vi "Example LV.vi"() -> ()   [LabVIEW 2020]
uses:
  <vilib>/Math Plots/3D Math Plots/3D Scatter/3D Scatter XCtrl/3D Scatter.xctl
  <vilib>/Utility/sysdir.llb/System Directory Type.ctl
  Sources/_Helpers/Tiff Page Details.ctl
  <vilib>/Analysis/1siggen.llb/Ramp Pattern by Samples.vi
  <vilib>/Math Plots/3D Math Plots/3D Scatter/3D Scatter Datatype/Public/Plot Helper (Matrix).vi
  Sources/TIFF Writer/TIFF Writer.lvclass
  Sources/LV Tiff.lvlib
  Sources/TIFF Reader/TIFF Reader.lvclass
  <vilib>/Analysis/NI_AALBase.lvlib
  <vilib>/Math Plots/3D Math Plots/3D Scatter/3D Scatter Datatype/3D Scatter Datatype.lvclass
panel:
  out "size(s)":i32
  out "3D Scatter":refnum<class "3D Plot Datatype.lvclass">[](xcontrol)
  out "Deflate":picture
  out "JPEG":picture
  out "Raw Picture":picture
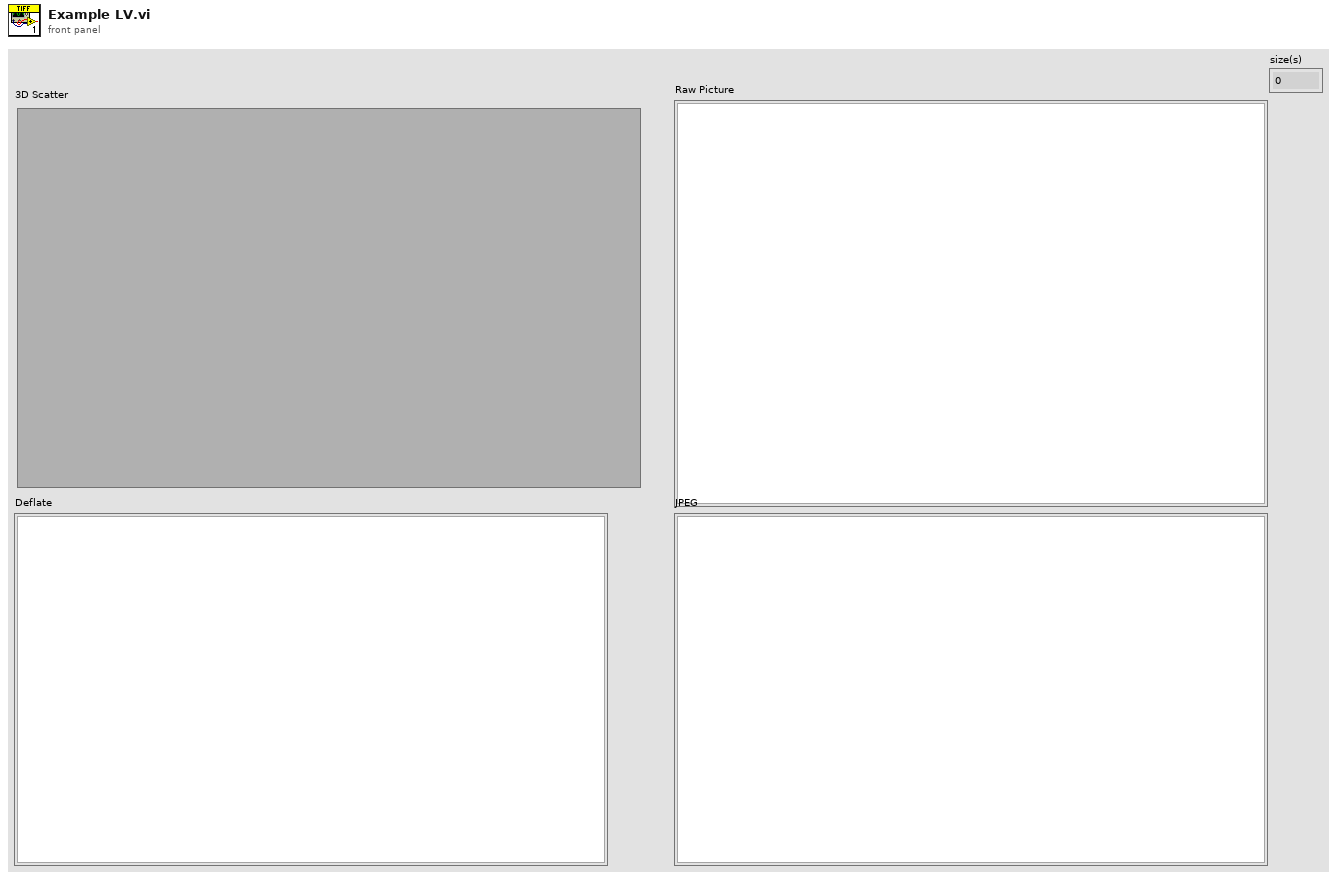
[diagram p1: front panel]
types:
  T1 = enum16{"open", "replace", "create", "open or create", "replace or create", "replace or create with confirmation"}
  T2 = typedef "System Directory Type.ctl" = i32
  T3 = typedef "imagedata.ctl" = cluster{"image type":i32, "image depth":i32, "image":u8[], "mask":u8[], "colors":u32[], "Rectangle":cluster{"left":i16, "top":i16, "right":i16, "bottom":i16}}
  T4 = typedef "LV Tiff.lvlib/Tiff Page Details.ctl" = cluster{"ImageDescription":string, "XResolution":dbl, "YResolution":dbl, "ResolutionUnit":enum16{"None", "Inch", "Centimeter"}, "PhotometricInterpretation":u16, "Compression":enum16{"None", "Deflate", "JPEG"}, "PageName":string, "DocumentName":string}
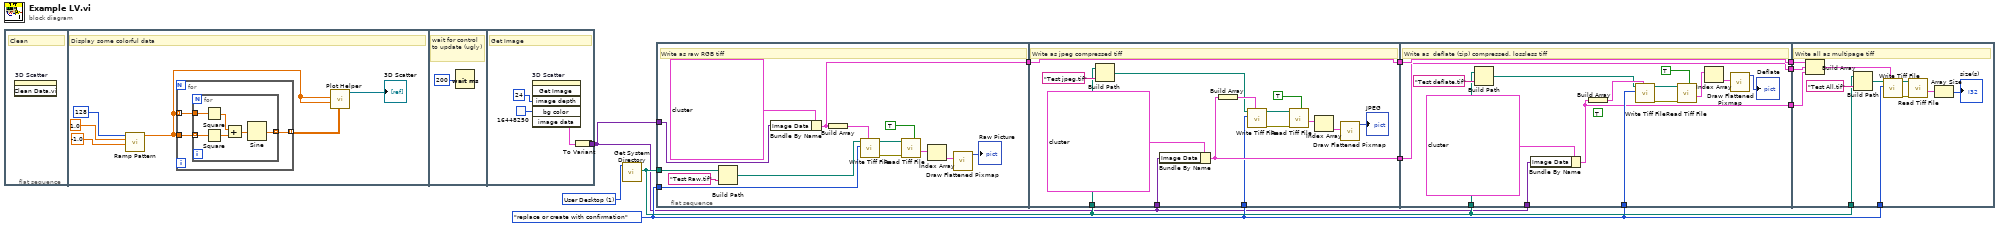
[diagram p0: block diagram]
diagram:
  w2 = T1."replace or create with confirmation" ("operation (replace)")
  w10 = T2 1 items=["User Home"=0, "User Desktop"=1, "User Documents"=2, "User Application Data"=3, "User Preferences"=4, "User Temporary"=5, "Public Documents"=6, "Public Application Data"=7, "Public Preferences"=8, "Public Cache"=13, "System Core Libraries"=9, "System Installed Libraries"=10, "Application Files"=11, "Boot Volume Root"=12] ("system directory type")
  n1 = flat-sequence {
    tunnel: [w27] -> w1
    frame #0 {
      # "Clean"
      n2 = invoke on="3D Scatter" class="3D Scatter (strict)" method="Clean Data.vi"() -> ()  [unwired: 3 in, 3 out]
    }
    frame #1 {
      # "Display some colorful data"
      n3 = call-poly <vilib>:"Ramp Pattern.vi"("start"=-1.0, "end"=1.0, "samples"=128) -> ("Ramp Pattern"=w12:dbl[])  [unwired: 7 in, 1 out]
      n4 = for {
        tunnel: [w19] -> w11 mode=indexing
        tunnel: w12 -> [w18] mode=indexing
        tunnel: w12 -> [w17]
        n5 = for {
          tunnel: [w25] -> w19 mode=indexing
          tunnel: w18 -> [w22]
          tunnel: w17 -> [w21] mode=indexing
          n6 = Square(x=w22) -> (x^2=w23:dbl)
          n7 = Square(x=w21) -> (x^2=w24:dbl)
          n8 = Add(x=w23, y=w24) -> (x+y=w20:dbl)
          n9 = Sine(x=w20) -> (sin(x)=w25:dbl)
        }
      }
      n10 = call-poly <vilib>:"Plot Helper.vi"("z matrix"=w11, "y vector"=w12, "x vector"=w12) -> ("3D Plot lvclass Array out"=→"3D Scatter":refnum<class "3D Plot Datatype.lvclass">[])  [unwired: 3 in, 5 out]
    }
    frame #2 {
      # "wait for control to update (ugly)"
      n11 = Wait (ms)(milliseconds to wait=u32 200) -> ()  [unwired: 1 out]
    }
    frame #3 {
      # "Get Image"
      n12 = invoke on="3D Scatter" class="3D Scatter (strict)" method="Get Image"("image depth"=24 ("Image Depth"), "bg color"=u32 16448250 ("Background Color")) -> ("image data"=w28:T3)  [unwired: 4 in, 5 out]
      n13 = To Variant(anything=w28) -> (Variant=w27:variant)
    }
  }
  n14 = call <vilib>:"Get System Directory.vi"("system directory type"=w10) -> ("system directory"=w8:path)  [unwired: 10 in]
  n15 = flat-sequence {
    tunnel: w2 -> [w38]
    tunnel: w1 -> [w32]
    tunnel: w8 -> [w36]
    tunnel: [w31] -> w5
    tunnel: w1 -> [w49]
    tunnel: w8 -> [w48]
    tunnel: [w47] -> w6
    tunnel: w5 -> [w47]
    tunnel: [w46] -> w3
    tunnel: w2 -> [w45]
    tunnel: w2 -> [w68]
    tunnel: w8 -> [w65]
    tunnel: w1 -> [w64]
    tunnel: [w63] -> w9
    tunnel: [w61] -> w7
    tunnel: w6 -> [w61]
    tunnel: [w60] -> w4
    tunnel: w3 -> [w60]
    tunnel: w9 -> [w85]
    tunnel: w8 -> [w86]
    tunnel: w2 -> [w79]
    tunnel: w7 -> [w77]
    tunnel: w4 -> [w76]
    frame #0 {
      # "Write as raw RGB tiff"
      n16 = Build Path(base path=w36, name or relative path="Test Raw.tif") -> (appended path=w37:path)
      n17 = Bundle By Name(cluster=cluster{"Image Data":variant, "Details":T4} {"Image Data"=variant, "Details"={"ImageDescription"="", "XResolution"=0.0, "YResolution"=0.0, "ResolutionUnit"=enum."Inch", "PhotometricInterpretation"=2, "Compression"=enum."None", "PageName"="", "DocumentName"=""}} ("Cluster"), "Image Data"=w32) -> (w31:cluster{"Image Data":variant, "Details":T4})
      n18 = Build Array(w31) -> (w33:cluster{"Image Data":variant, "Details":T4}[])
      n19 = call "Write Tiff File.vi"("Pages"=w33, "operation (replace)"=w38, "Path"=w37) -> ("error out"=w41:errorcluster, "path"=w34:path)  [unwired: 7 in]
      n20 = call "Read Tiff File.vi"("Create Flattened Images (24 Bit only)"=TRUE, "error in (no error)"=w41, "Path"=w34) -> ("Flattened Images"=w42:T3[])  [unwired: 5 in, 3 out]
      n21 = Index Array(array=w42) -> (element=w43:T3)  [unwired: 1 in]
      n22 = call <vilib>:"Draw Flattened Pixmap.vi"("image data"=w43) -> ("new picture"=→"Raw Picture":picture)  [unwired: 8 in]
    }
    frame #1 {
      # "Write as jpeg compressed tiff"
      n23 = Build Path(base path=w48, name or relative path="Test jpeg.tif") -> (appended path=w56:path)
      n24 = Bundle By Name(cluster=cluster{"Image Data":variant, "Details":T4} {"Image Data"=variant, "Details"={"ImageDescription"="", "XResolution"=0.0, "YResolution"=0.0, "ResolutionUnit"=enum."Inch", "PhotometricInterpretation"=6, "Compression"=enum."JPEG", "PageName"="", "DocumentName"=""}} ("Cluster"), "Image Data"=w49) -> (w46:cluster{"Image Data":variant, "Details":T4})
      n25 = Build Array(w46) -> (w57:cluster{"Image Data":variant, "Details":T4}[])
      n26 = call "Write Tiff File.vi"("Pages"=w57, "operation (replace)"=w45, "Path"=w56) -> ("error out"=w50:errorcluster, "path"=w51:path)  [unwired: 7 in]
      n27 = call "Read Tiff File.vi"("Create Flattened Images (24 Bit only)"=TRUE, "error in (no error)"=w50, "Path"=w51) -> ("Flattened Images"=w53:T3[])  [unwired: 5 in, 3 out]
      n28 = Index Array(array=w53) -> (element=w54:T3)  [unwired: 1 in]
      n29 = call <vilib>:"Draw Flattened Pixmap.vi"("image data"=w54) -> ("new picture"=→"JPEG":picture)  [unwired: 8 in]
    }
    frame #2 {
      (unwired) TRUE ("Create Flattened Images (24 Bit only)")
      # "Write as  deflate (zip) compressed, lossless tiff"
      n30 = Build Path(base path=w65, name or relative path="Test deflate.tif") -> (appended path=w62:path)
      n31 = Bundle By Name(cluster=cluster{"Image Data":variant, "Details":T4} {"Image Data"=variant, "Details"={"ImageDescription"="", "XResolution"=0.0, "YResolution"=0.0, "ResolutionUnit"=enum."Inch", "PhotometricInterpretation"=2, "Compression"=enum."Deflate", "PageName"="", "DocumentName"=""}} ("Cluster"), "Image Data"=w64) -> (w63:cluster{"Image Data":variant, "Details":T4})
      n32 = Build Array(w63) -> (w75:cluster{"Image Data":variant, "Details":T4}[])
      n33 = call "Write Tiff File.vi"("Pages"=w75, "operation (replace)"=w68, "Path"=w62) -> ("error out"=w70:errorcluster, "path"=w71:path)  [unwired: 7 in]
      n34 = call "Read Tiff File.vi"("Create Flattened Images (24 Bit only)"=TRUE, "error in (no error)"=w70, "Path"=w71) -> ("Flattened Images"=w72:T3[])  [unwired: 5 in, 3 out]
      n35 = Index Array(array=w72) -> (element=w73:T3)  [unwired: 1 in]
      n36 = call <vilib>:"Draw Flattened Pixmap.vi"("image data"=w73) -> ("new picture"=→"Deflate":picture)  [unwired: 8 in]
    }
    frame #3 {
      # "Write all as multipage tiff"
      n37 = Build Array(w77, w76, w85) -> (w80:cluster{"Image Data":variant, "Details":T4}[])
      n38 = Build Path(base path=w86, name or relative path="Test All.tif") -> (appended path=w78:path)
      n39 = call "Write Tiff File.vi"("Pages"=w80, "operation (replace)"=w79, "Path"=w78) -> ("error out"=w82:errorcluster, "path"=w81:path)  [unwired: 7 in]
      n40 = call "Read Tiff File.vi"("error in (no error)"=w82, "Path"=w81) -> ("Flattened Images"=w83:T3[])  [unwired: 6 in, 3 out]
      n41 = Array Size(array=w83) -> (size(s)=→"size(s)":i32)
    }
  }
